vi "5-dist.vi"(0 "Poisson (m)":T1, 1 "k max":i16) -> (3 "F(k max)":dbl, 8 "f(0 à k max)":dbl[](array[numeric]), 10 "F(0 à k max)":dbl[](array[numeric]))   [LabVIEW 2010, in "lv_02.lvlib"]
uses:
  lv_02.lvlib
  p_5E5_LPoi.ctl
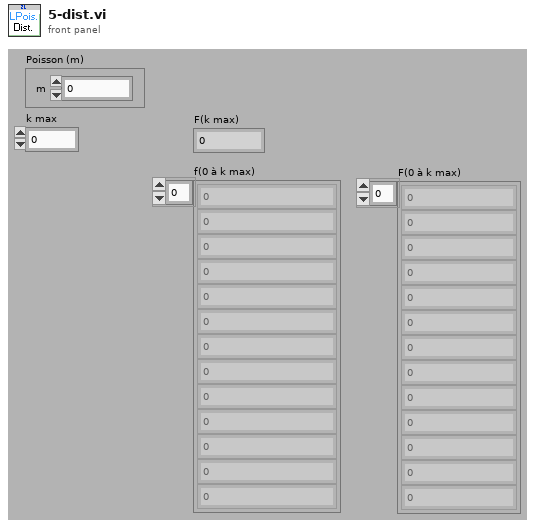
[diagram p1: front panel]
types:
  T1 = typedef "lv_02.lvlib/p_5E5_LPoi.ctl" = cluster{"m":dbl}
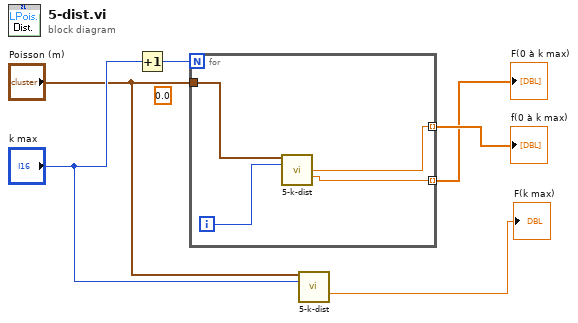
[diagram p0: block diagram]
diagram:
  (unwired) 0.0
  n1 = Increment(x="k max") -> (x+1=w6:i16)
  n2 = for {
    N: w6 -> [_]
    tunnel: [w10] -> w5 mode=indexing
    tunnel: [w9] -> w4 mode=indexing
    tunnel: "Poisson (m)" -> [w7]
    i -> [w8]
    n3 = call "5-k-dist.vi"("Loi de Poisson"=w7, "k"=w8) -> ("p(X=k)"=w10:dbl, "F(X<=k)"=w9:dbl)  [unwired: 9 in, 3 out]
  }
  "f(0 à k max)" <- w5
  "F(0 à k max)" <- w4
  n4 = call "5-k-dist.vi"("Loi de Poisson"="Poisson (m)", "k"="k max") -> ("F(X<=k)"=→"F(k max)":dbl)  [unwired: 9 in, 4 out]
